vi "Pfeiffer_Driver_Core.vi"(0 "Command":string, 1 "Write/Read":bool, 2 "Port":i32(ring) items=["COM 1", "COM 2", "COM 3", "COM 4", "COM 5", "COM 6", "COM 7", "COM 8", "COM 9", "LPT 1", "LPT 2", "LPT 3", "LPT 4"], 12 "Timeout [ms]":u32=600 min=1 max=40000 step=1, 13 "Retry (3)":i32=3 min=1 max=20000 step=1) -> (8 "String Out":string, 10 "NAK":bool, 15 "Error":bool)   [LabVIEW 2010]
doc: "VI runs with TPG 252 / TPG 261 / TPG 262 !"
panel:
  out "?":i32
  in  "ENQ [\\05]":string="\u0005"
  in  "NAK [\\15]":string="\u0015"
  in  "ACK [\\06]":string="\u0006"
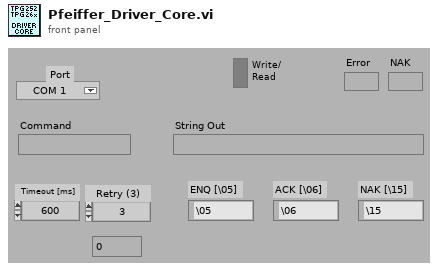
[diagram p1: front panel]
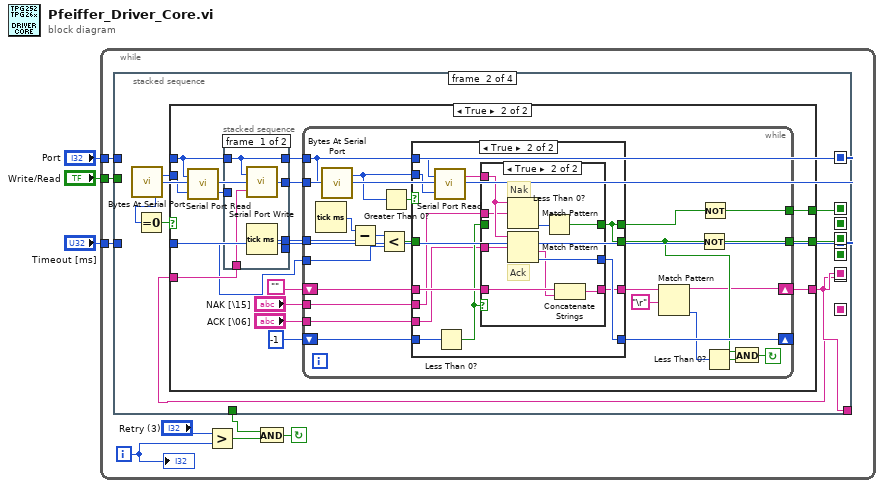
[diagram p0: block diagram]
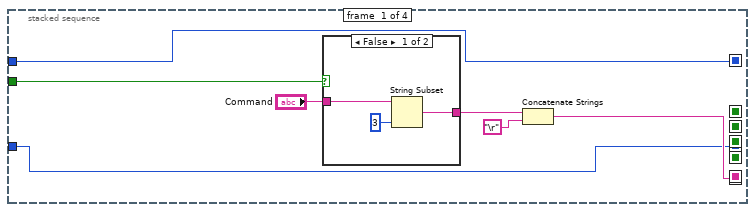
[diagram p2: hidden frame]
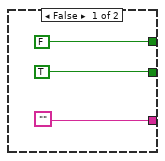
[diagram p4: hidden frame]
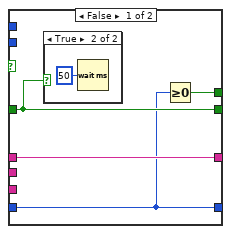
[diagram p5: hidden frame]
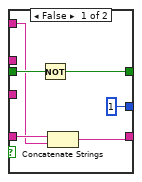
[diagram p7: hidden frame]
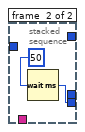
[diagram p8: hidden frame]
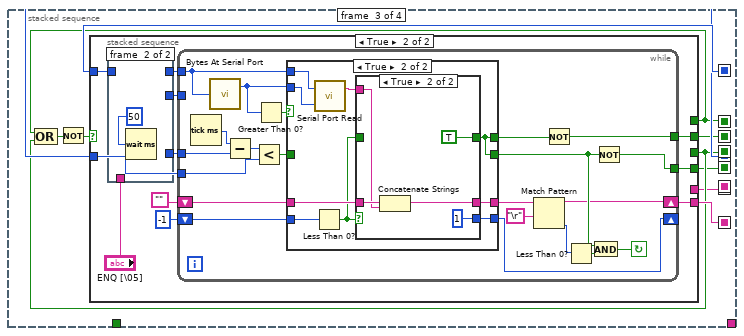
[diagram p9: hidden frame]
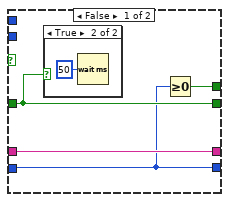
[diagram p11: hidden frame]
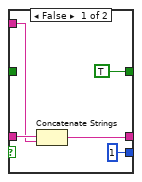
[diagram p13: hidden frame]
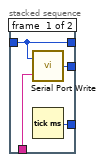
[diagram p14: hidden frame]
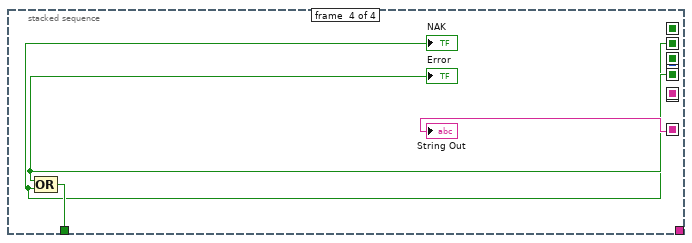
[diagram p15: hidden frame]
diagram:
  n1 = while {
    tunnel: "Write/Read" -> [w4]
    tunnel: "Timeout [ms]" -> [w10]
    tunnel: "Port" -> [w11]
    i -> [w8]
    stop <- w5 continue-if-true
    n2 = stacked-sequence {
      seq-local: [w13 _ _ _] -> [_ w29 _ _]
      seq-local: [w12 _ _ _] -> [_ w28 _ _]
      seq-local: [w18 _ _ _] -> [_ w27 _ _]
      seq-local: [_ w29 _ _] -> [_ _ w119 _]
      seq-local: [_ w28 _ _] -> [_ _ w118 _]
      seq-local: [_ w31 _ _] -> [_ _ w111 _]
      seq-local: [_ w23 _ _] -> [_ _ w113 _]
      seq-local: [_ w24 _ _] -> [_ _ w112 _]
      seq-local: [_ _ w117 _] -> [_ _ _ w184]
      seq-local: [_ _ w110 _] -> [_ _ _ w185]
      seq-local: [_ _ w116 _] -> [_ _ _ w186]
      tunnel: w11 -> [w13 _ _ _]
      tunnel: w10 -> [w12 _ _ _]
      tunnel: w4 -> [w17 _ _ _]
      tunnel: [_ w31 _ _] -> _
      tunnel: [_ _ _ w187] -> w6
      frame #0 {
        n3 = case shown="False" w17 {
          tunnel: "Command" -> [w21 w22]
          tunnel: [w20 w22] -> w16
          frame False {
            n4 = String Subset(string=w21, length (rest)=u8 3 ("t")) -> (substring=w20:string)  [unwired: 1 out]
          }
          frame True {
          }
        }
        n5 = Concatenate Strings(w16, "\r") -> (w18:string)
      }
      frame #1 {
        n6 = call <vilib>:"Bytes At Serial Port.vi"("port number"=w29) -> ("byte count"=w30:u32, "error code"=w25:i32)
        n7 = Equal To 0?(x=w25) -> (x = 0?=w26:bool)
        n8 = case shown="True" w26 {
          tunnel: [FALSE w49] -> w23
          tunnel: [TRUE w48] -> w24
          tunnel: w27 -> [_ w44]
          tunnel: w28 -> [_ w43]
          tunnel: w29 -> [_ w42]
          tunnel: w30 -> [_ w41]
          tunnel: ["" w37] -> w31
          frame False {
          }
          frame True {
            n9 = call <vilib>:"Serial Port Read.vi"("requested byte count"=w41, "port number"=w42) -> ("error code"=w38:i32)  [unwired: 1 out]
            n10 = stacked-sequence {
              tunnel: w42 -> [w105 _]
              tunnel: w44 -> [w107 _]
              tunnel: [w106 _] -> w36
              tunnel: w38 -> [_ _]
              tunnel: [w105 _] -> w39
              tunnel: [w104 _] -> w40
              tunnel: [_ w108] -> _
              frame #0 {
                n11 = call <vilib>:"Serial Port Write.vi"("string to write"=w107, "port number"=w105) -> ("error code"=w106:i32)
                n12 = Tick Count (ms)() -> (millisecond timer value=w104:u32)
              }
              frame #1 {
                n13 = Wait (ms)(milliseconds to wait=u32 50) -> (millisecond timer value=w108:u32)
              }
            }
            n14 = while {
              tunnel: "ACK [\\06]" -> [w55]
              tunnel: "NAK [\\15]" -> [w56]
              tunnel: [w58] -> w49
              tunnel: [w60] -> w48
              shift-left: -1 -> [w64]
              shift-right: [w63] -> _
              shift-left: "" -> [w65]
              shift-right: [w53] -> w37
              tunnel: w40 -> [w66]
              tunnel: w43 -> [w71]
              tunnel: w39 -> [w69]
              tunnel: w36 -> [_]
              stop <- w62 continue-if-true
              n15 = Tick Count (ms)() -> (millisecond timer value=w67:u32)
              n16 = call <vilib>:"Bytes At Serial Port.vi"("port number"=w69) -> ("byte count"=w57:u32)  [unwired: 1 out]
              n17 = Subtract(x=w67, y=w66) -> (x-y=w72:u32)
              n18 = Less?(x=w72, y=w71) -> (x < y?=w68:bool)
              n19 = Greater Than 0?(x=w57) -> (x > 0?=w70:bool)
              n20 = case shown="True" w70 {
                tunnel: w69 -> [_ w88]
                tunnel: w57 -> [_ w87]
                tunnel: w68 -> [w75 _]
                tunnel: w65 -> [w76 w84]
                tunnel: w64 -> [w73 w85]
                tunnel: [w73 w83] -> w63
                tunnel: [w76 w82] -> w54
                tunnel: [w75 w78] -> w61
                tunnel: [w74 w78] -> w59
                tunnel: w56 -> [_ w80]
                tunnel: w55 -> [_ w79]
                frame False {
                  n21 = case shown="True" w75 {
                    frame False {
                    }
                    frame True {
                      n22 = Wait (ms)(milliseconds to wait=u32 50) -> ()  [unwired: 1 out]
                    }
                  }
                  n23 = Greater Or Equal To 0?(x=w73) -> (x >= 0?=w74:bool)
                }
                frame True {
                  n24 = call <vilib>:"Serial Port Read.vi"("requested byte count"=w87, "port number"=w88) -> ("string read"=w86:string)  [unwired: 1 out]
                  n25 = Less Than 0?(x=w85) -> (x < 0?=w81:bool)
                  n26 = case shown="True" w81 {
                    tunnel: w86 -> [w89 w100]
                    tunnel: w84 -> [w94 w103]
                    tunnel: [1 w102] -> w83
                    tunnel: [w93 w101] -> w82
                    tunnel: [w90 w98] -> w78
                    tunnel: w81 -> [w91 _]
                    tunnel: w80 -> [_ w96]
                    tunnel: w79 -> [_ w95]
                    frame False {
                      n27 = Not(x=w91) -> (.not. x?=w90:bool)
                      n28 = Concatenate Strings(w94, w89) -> (w93:string)
                    }
                    frame True {
                      # "Ack"
                      # "Nak"
                      n29 = Match Pattern(string=w100, regular expression=w96) -> (offset past match=w99:i32)  [unwired: 4 out]
                      n30 = Match Pattern(string=w100, regular expression=w95) -> (after substring=w97:string, offset past match=w102:i32)  [unwired: 3 out]
                      n31 = Less Than 0?(x=w99) -> (x < 0?=w98:bool)
                      n32 = Concatenate Strings(w103, w97) -> (w101:string)
                    }
                  }
                }
              }
              n33 = Match Pattern(string=w54, regular expression="\r") -> (before substring=w53:string, offset past match=w50:i32)  [unwired: 3 out]
              n34 = Not(x=w61) -> (.not. x?=w60:bool)
              n35 = Not(x=w59) -> (.not. x?=w58:bool)
              n36 = Less Than 0?(x=w50) -> (x < 0?=w51:bool)
              n37 = And(x=w61, y=w51) -> (x .and. y?=w62:bool)
            }
          }
        }
      }
      frame #2 {
        n38 = Compound Arithmetic op=OR(w113, w112) -> (w115:bool)
        n39 = Not(x=w115) -> (.not. x?=w114:bool)
        n40 = case shown="True" w114 {
          tunnel: w118 -> [_ w132]
          tunnel: w119 -> [_ w131]
          tunnel: [w122 w125] -> w117
          tunnel: [w121 w124] -> w110
          tunnel: [w120 w123] -> w116
          tunnel: w113 -> [w122 _]
          tunnel: w112 -> [w121 _]
          tunnel: w111 -> [w120 _]
          frame False {
          }
          frame True {
            n41 = stacked-sequence {
              tunnel: w131 -> [w180 _]
              tunnel: "ENQ [\\05]" -> [w182 _]
              tunnel: [w181 _] -> w128
              tunnel: [w180 _] -> w129
              tunnel: [w179 _] -> w130
              frame #0 {
                n42 = call <vilib>:"Serial Port Write.vi"("string to write"=w182, "port number"=w180) -> ("error code"=w181:i32)
                n43 = Tick Count (ms)() -> (millisecond timer value=w179:u32)
              }
              frame #1 {
                n44 = Wait (ms)(milliseconds to wait=u32 50) -> ()  [unwired: 1 out]
              }
            }
            n45 = while {
              tunnel: [w134] -> w124
              tunnel: [w135] -> w125
              shift-left: -1 -> [w146]
              shift-right: [w145] -> _
              shift-left: "" -> [w147]
              shift-right: [w139] -> w123
              tunnel: w130 -> [w148]
              tunnel: w132 -> [w153]
              tunnel: w129 -> [w151]
              tunnel: w128 -> [_]
              stop <- w144 continue-if-true
              n46 = Tick Count (ms)() -> (millisecond timer value=w149:u32)
              n47 = call <vilib>:"Bytes At Serial Port.vi"("port number"=w151) -> ("byte count"=w141:u32)  [unwired: 1 out]
              n48 = Subtract(x=w149, y=w148) -> (x-y=w154:u32)
              n49 = Less?(x=w154, y=w153) -> (x < y?=w150:bool)
              n50 = Greater Than 0?(x=w141) -> (x > 0?=w152:bool)
              n51 = case shown="True" w152 {
                tunnel: w151 -> [_ w168]
                tunnel: w141 -> [_ w167]
                tunnel: w150 -> [w157 _]
                tunnel: w147 -> [w158 w164]
                tunnel: w146 -> [w155 w165]
                tunnel: [w155 w163] -> w145
                tunnel: [w158 w162] -> w140
                tunnel: [w157 w160] -> w143
                tunnel: [w156 w160] -> w142
                frame False {
                  n52 = case shown="True" w157 {
                    frame False {
                    }
                    frame True {
                      n53 = Wait (ms)(milliseconds to wait=u32 50) -> ()  [unwired: 1 out]
                    }
                  }
                  n54 = Greater Or Equal To 0?(x=w155) -> (x >= 0?=w156:bool)
                }
                frame True {
                  n55 = Less Than 0?(x=w165) -> (x < 0?=w161:bool)
                  n56 = call <vilib>:"Serial Port Read.vi"("requested byte count"=w167, "port number"=w168) -> ("string read"=w166:string)  [unwired: 1 out]
                  n57 = case shown="True" w161 {
                    tunnel: w166 -> [w170 w176]
                    tunnel: w164 -> [w173 w178]
                    tunnel: [1 1] -> w163
                    tunnel: [w172 w177] -> w162
                    tunnel: [TRUE TRUE] -> w160
                    tunnel: w161 -> [_ _]
                    frame False {
                      n58 = Concatenate Strings(w173, w170) -> (w172:string)
                    }
                    frame True {
                      n59 = Concatenate Strings(w178, w176) -> (w177:string)
                    }
                  }
                }
              }
              n60 = Match Pattern(string=w140, regular expression="\r") -> (before substring=w139:string, offset past match=w136:i32)  [unwired: 3 out]
              n61 = Not(x=w142) -> (.not. x?=w135:bool)
              n62 = Less Than 0?(x=w136) -> (x < 0?=w137:bool)
              n63 = And(x=w143, y=w137) -> (x .and. y?=w144:bool)
              n64 = Not(x=w143) -> (.not. x?=w134:bool)
            }
          }
        }
      }
      frame #3 {
        n65 = Compound Arithmetic op=OR(w185, w184) -> (w187:bool)
        "Error" <- w185
        "NAK" <- w184
        "String Out" <- w186
      }
    }
    n66 = Greater?(x="Retry (3)", y=w8) -> (0:w7:bool)
    n67 = And(x=w6, y=w7) -> (x .and. y?=w5:bool)
    "?" <- w8
  }
